vi "Auto Pickup Global.vi"() -> ()   [LabVIEW 2013]
panel:
  in  "Enable Auto Pickup":bool
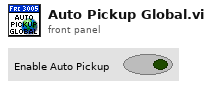
[diagram p1: front panel]
diagram:
